vi "Begin.vi"() -> (0 "error out":errorcluster)   [LabVIEW 2013]
doc: "Called before other user functions, this VI is expected to open initial I/O refnums, load in file data, and do all program initialization. Notice that the <B>error out</B> terminal is simply used for data flow. Wiring it to other structures or subVIs ensures that this VI runs first."
uses:
  <vilib>/Rock Robotics/WPI/Joystick/WPI_JoystickDeviceEnum.ctl
  <vilib>/Rock Robotics/SystemInterfaces/Typedef/FPGA_TypedefDigitalModule.ctl
  <vilib>/Rock Robotics/SystemInterfaces/DIO/FPGA_DIOChannel.ctl
  <vilib>/Rock Robotics/SystemInterfaces/DIO/FPGA_DIORelayChannel.ctl
  <vilib>/Rock Robotics/SystemInterfaces/Typedef/FPGA_TypedefSolenoidModule.ctl
  <vilib>/Rock Robotics/WPI/Solenoid/WPI_SolenoidChannel.ctl
  <vilib>/Rock Robotics/SystemInterfaces/DIO/FPGA_DIOPWMChannel.ctl
  <vilib>/Rock Robotics/WPI/Encoder/WPI_EncoderType.ctl
  <vilib>/Rock Robotics/WPI/Solenoid/WPI_SolenoidValue.ctl
  <vilib>/Rock Robotics/WPI/Camera/WPI_CameraImageSize.ctl
  <vilib>/Rock Robotics/WPI/Camera/WPI_CameraWhite Balance Values.ctl
  <vilib>/Rock Robotics/WPI/Camera/WPI_CameraExposure Values.ctl
  <vilib>/Rock Robotics/WPI/Camera/WPI_CameraFrameRate.ctl
  <vilib>/Rock Robotics/WPI/Solenoid/WPI_SolenoidOpenDouble.vi
  <vilib>/Rock Robotics/WPI/Solenoid/WPI_SolenoidSetEnum.vi
  <vilib>/Rock Robotics/WPI/Counter/WPI_CounterDigitalInputToDigitalSource.vi
  <vilib>/Rock Robotics/WPI/RobotDrive/WPI_RobotDriveOpen2MotorWithVictor.vi
  <vilib>/Rock Robotics/WPI/MotorControl/WPI_MotorControlOpen Jaguar.vi
  <vilib>/Rock Robotics/WPI/MotorControl/WPI_MotorControlOpen Victor.vi
  <vilib>/Rock Robotics/WPI/Compressor/WPI_CompressorGetSetRefNum.vi
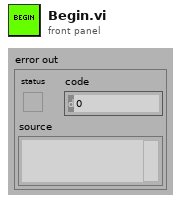
[diagram p1: front panel]
types:
  T1 = typedef "WPI_SolenoidValue.ctl" = enum16{"Off", "On", "Forward", "Reverse"}
  T2 = typedef "FPGA_DIOChannel.ctl" = enum8{"DIO 1", "DIO 2", "DIO 3", "DIO 4", "DIO 5", "DIO 6", "DIO 7", "DIO 8", "DIO 9", "DIO 10", "DIO 11", "DIO 12", "DIO 13", "DIO 14", "Invalid"}
  T3 = typedef "WPI_SolenoidChannel.ctl" = enum8{"Solenoid 1", "Solenoid 2", "Solenoid 3", "Solenoid 4", "Solenoid 5", "Solenoid 6", "Solenoid 7", "Solenoid 8", "Invalid"}
  T4 = typedef "FPGA_DIOPWMChannel.ctl" = enum8{"PWM 1", "PWM 2", "PWM 3", "PWM 4", "PWM 5", "PWM 6", "PWM 7", "PWM 8", "PWM 9", "PWM 10", "Invalid"}
  T5 = typedef "WPI_EncoderType.ctl" = enum16{"1x", "2x", "4x"}
  T6 = typedef "FPGA_TypedefSolenoidModule.ctl" = enum16{"Solenoid Module 1", "Solenoid Module 2"}
  T7 = typedef "FPGA_DIORelayChannel.ctl" = enum8{"Relay 1", "Relay 2", "Relay 3", "Relay 4", "Relay 5", "Relay 6", "Relay 7", "Relay 8", "Invalid"}
  T8 = typedef "WPI_JoystickDeviceEnum.ctl" = enum16{"USB 1", "USB 2", "USB 3", "USB 4", "Kinect 1", "Kinect 2"}
  T9 = typedef "FPGA_TypedefDigitalModule.ctl" = enum16{"Digital Module 1", "Digital Module 2"}
  T10 = typedef "WPI_CameraFrameRate.ctl" = u32
  T11 = typedef "WPI_CameraExposure Values.ctl" = enum16{"Auto", "Flicker-free 50 Hz", "Flicker-free 60 Hz", "Hold current"}
  T12 = typedef "WPI_CameraWhite Balance Values.ctl" = enum16{"Auto", "Fixed indoor", "Fixed outdoor 1", "Fixed outdoor 2", "Fixed fluorescent 1", "Fixed fluorescent 2", "Hold current"}
  T13 = typedef "WPI_CameraImageSize.ctl" = enum16{"640x480", "320x240", "160x120"}
  T14 = typedef "WPI_CameraDevRef.ctl" = cluster{"Camera Address":string, "CameraStatus":errorcluster, "Acquire Image Notifier":refnum<notifier>}
  T15 = typedef "WPI_DigitalInputDevRef.ctl" = cluster{"DevStatus":errorcluster, "DIO Channel":T2, "Digital Module":T9}
  T16 = typedef "WPI_MotorControlDeviceRef.ctl" = cluster{"DeviceStatus":errorcluster, "Type":enum16{"PWM", "CAN"}, "PWM":cluster{"Digital Module":T9, "PWM Channel":T4, "DeadBand":T17}, "CAN":cluster{"Device Number":u8, "Control Mode":T18, "Semaphore":T19, "Max Vout":dbl}, "Invert":bool, "TransformRef":T20, "InvTransformRef":T20}
  T17 = typedef "WPI_PWMDeadband.ctl" = cluster{"Name":string, "maxPositivePwm":i32, "minPositivePwm":i32, "centerPwm":i32, "maxNegativePwm":i32, "minNegativePwm":i32, "angularRange":u16}
  T18 = typedef "WPI_CANJaguar_ControlMode.ctl" = enum8{"Percent VBus", "Current", "Speed", "Position", "Voltage"}
  T19 = typedef "Semaphore RefNum" = refnum<k1>
  T20 = typedef "WPI_PWMTransform_ConPane.ctl" = refnum<vi>
  T21 = typedef "WPI_SolenoidDevRef.ctl" = cluster{"DevStatus":errorcluster, "Solenoid Module":T6, "Forward Solenoid Channel":T3, "Reverse Solenoid Channel":T3}
  T22 = typedef "FPGA_CounterEncoderSourceConvertionLVSourceType.ctl" = cluster{"DevStatus":errorcluster, "AnalogTriggerMode?":bool, "DigitalMode":cluster{"Digital Module":T9, "DIO Channel":T23}, "AnalogTriggerMode":cluster{"AnalogTriggerIndex":T24, "OutputType":T25}}
  T23 = typedef "FPGA_DIODigitalSourceChannel.ctl" = enum8{"DIO 1", "DIO 2", "DIO 3", "DIO 4", "DIO 5", "DIO 6", "DIO 7", "DIO 8", "DIO 9", "DIO 10", "DIO 11", "DIO 12", "DIO 13", "DIO 14", "Disabled"}
  T24 = typedef "FPGA_AnalogTriggerIndex.ctl" = enum8{"Trig 0", "Trig 1", "Trig 2", "Trig 3", "Trig 4", "Trig 5", "Trig 6", "Trig 7", "Invalid"}
  T25 = typedef "FPGA_AnalogTriggerOutType.ctl" = enum16{"InWindow", "TriggerState", "Rising", "Falling"}
  T26 = typedef "WPI_CompressorDevRef.ctl" = cluster{"DevStatus":errorcluster, "DigitalInputDevRef":T15, "RelayDevRef":T27}
  T27 = typedef "WPI_RelayDevRef.ctl" = cluster{"DevStatus":errorcluster, "Relay Channel":T7, "Digital Module":T9, "Relay Direction":T28}
  T28 = typedef "WPI_RelayDirection.ctl" = enum16{"Both directions", "Forward only", "Reverse only"}
  T29 = typedef "WPI_RobotDriveDevRef.ctl" = cluster{"DevStatus":errorcluster, "Motors[]":T16[], "Square Inputs":bool, "Max Output":dbl, "Isochronous":bool}
  T30 = typedef "WPI_EncoderDevRef.ctl" = cluster{"DevStatus":errorcluster, "EncoderIndex":T31, "CounterIndex":T32, "DistancePerCount":dbl, "Decoding Type":T5}
  T31 = typedef "FPGA_EncoderIdx.ctl" = enum8{"Enc 0", "Enc 1", "Enc 2", "Enc 3", "Invalid"}
  T32 = typedef "FPGA_CounterCtrSystemIndex.ctl" = enum8{"Ctr 0", "Ctr 1", "Ctr 2", "Ctr 3", "Ctr 4", "Ctr 5", "Ctr 6", "Ctr 7", "Invalid"}
  T33 = typedef "WPI_JoystickDevRef.ctl" = cluster{"Device":T8}
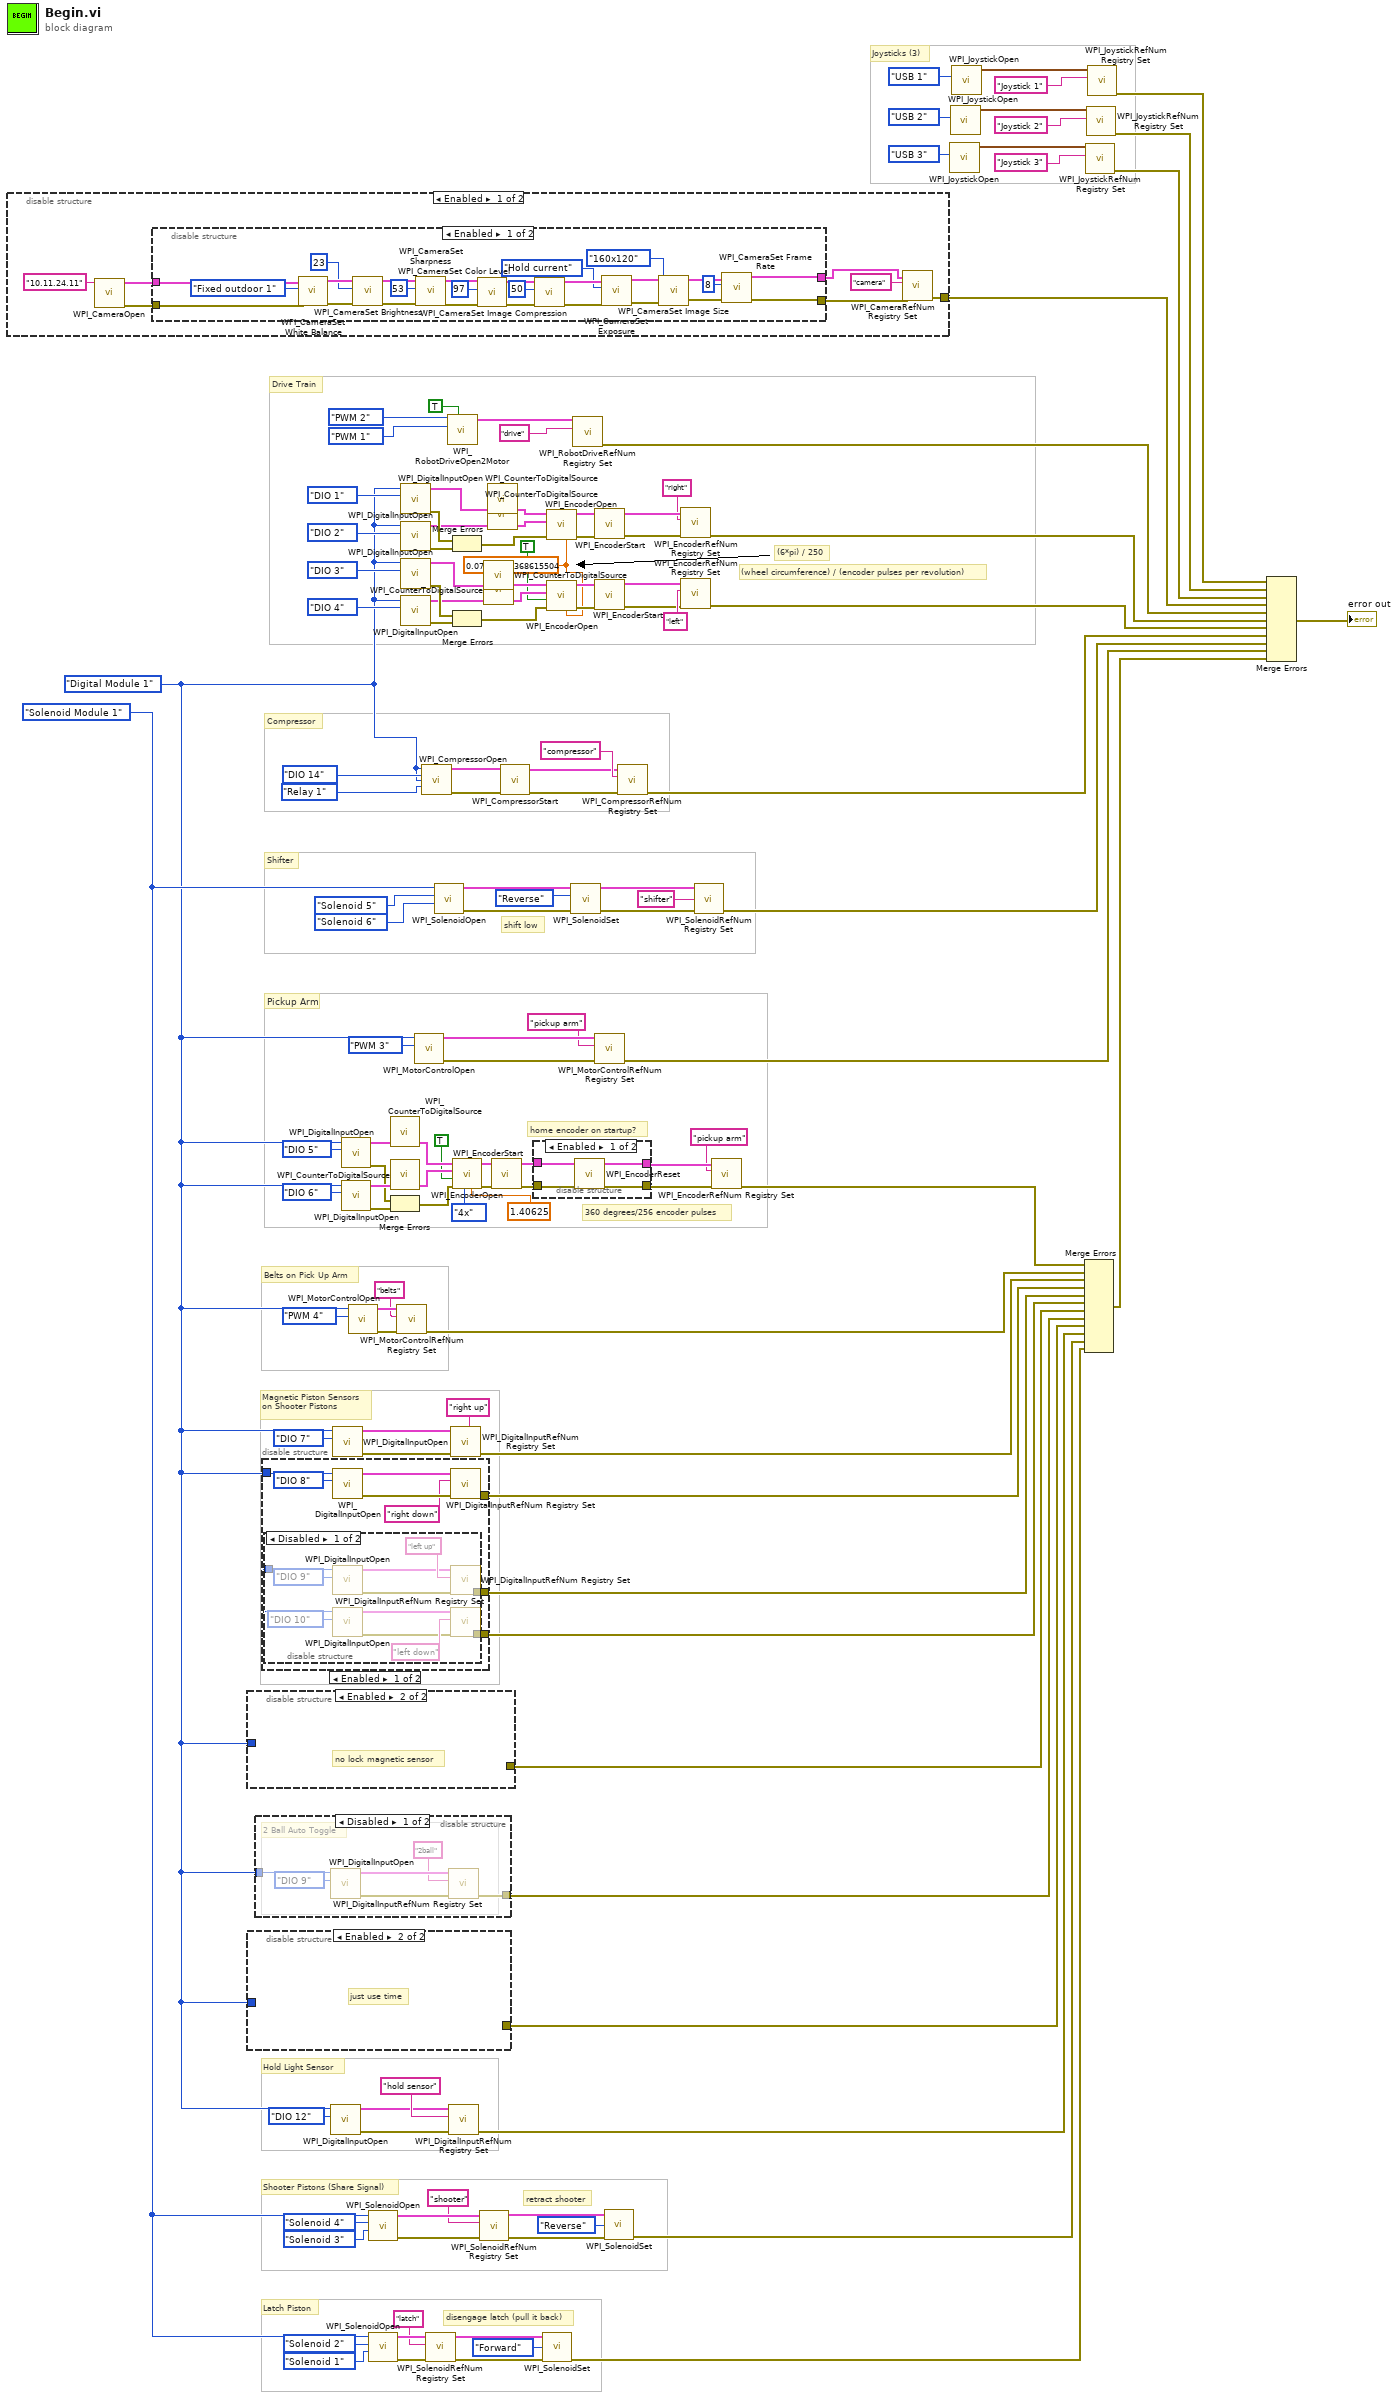
[diagram p0: block diagram]
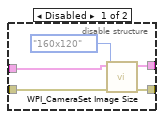
[diagram p4: hidden frame]
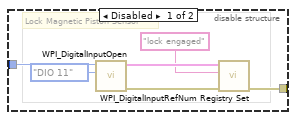
[diagram p6: hidden frame]
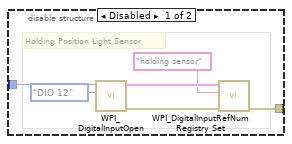
[diagram p9: hidden frame]
diagram:
  w80 = 0.07539822368615504 ("DistancePerCount")
  w23 = FPGA_TypedefSolenoidModule."Solenoid Module 1" ("Solenoid Module (Module 1)")
  w12 = FPGA_TypedefDigitalModule."Digital Module 1" ("Digital Module (Module 1)")
  # "retract shooter"
  # "disengage latch (pull it back)"
  # "360 degrees/256 encoder pulses"
  # "Hold Light Sensor"
  # "Joysticks (3)"
  # "Latch Piston"
  # "Shooter Pistons (Share Signal)"
  # "Magnetic Piston Sensors\non Shooter Pistons"
  # "Belts on Pick Up Arm"
  # "Pickup Arm"
  # "home encoder on startup?"
  # "Shifter"
  # "Compressor"
  # "Drive Train"
  # "shift low"
  # "(wheel circumference) / (encoder pulses per revolution)"
  # "(6*pi) / 250"
  n1 = disable-structure shown="Enabled" {
    disable-tunnel: [w143 _] -> w124
    frame Enabled {
      n2 = call <vilib>:"WPI_CameraOpen.vi"("Camera Address"="10.11.24.11") -> ("error out"=w138:errorcluster, "CameraDevRef"=w140:T14)  [unwired: 9 in]
      n3 = disable-structure shown="Enabled" {
        disable-tunnel: w140 -> [w167 w173]
        disable-tunnel: [w145 w172] -> w139
        disable-tunnel: w138 -> [w154 w171]
        disable-tunnel: [w144 w170] -> w137
        frame Enabled {
          n4 = call <vilib>:"WPI_CameraSet White Balance.vi"("error in (no error)"=w154, "White Balance"=WPI_CameraWhite_Balance_Values."Fixed outdoor 1", "CameraDevRef"=w167) -> ("error out"=w155:errorcluster, "CameraDevRef Out"=w166:T14)  [unwired: 7 in]
          n5 = call <vilib>:"WPI_CameraSet Brightness.vi"("error in (no error)"=w155, "Brightness"=23, "CameraDevRef"=w166) -> ("error out"=w156:errorcluster, "CameraDevRef Out"=w165:T14)  [unwired: 7 in]
          n6 = call <vilib>:"WPI_CameraSet Sharpness.vi"("error in (no error)"=w156, "Sharpness"=53, "CameraDevRef"=w165) -> ("error out"=w157:errorcluster, "CameraDevRef Out"=w164:T14)  [unwired: 7 in]
          n7 = call <vilib>:"WPI_CameraSet Color Level.vi"("error in (no error)"=w157, "Color Level"=97, "CameraDevRef"=w164) -> ("error out"=w158:errorcluster, "CameraDevRef Out"=w163:T14)  [unwired: 7 in]
          n8 = call <vilib>:"WPI_CameraSet Image Compression.vi"("error in (no error)"=w158, "Compression"=50, "CameraDevRef"=w163) -> ("error out"=w169:errorcluster, "CameraDevRef Out"=w168:T14)  [unwired: 7 in]
          n9 = call <vilib>:"WPI_CameraSet Exposure.vi"("error in (no error)"=w169, "Exposure"=WPI_CameraExposure_Values."Hold current", "CameraDevRef"=w168) -> ("error out"=w159:errorcluster, "CameraDevRef Out"=w162:T14)  [unwired: 7 in]
          n10 = call <vilib>:"WPI_CameraSet Image Size.vi"("error in (no error)"=w159, "Image Size"=WPI_CameraImageSize."160x120", "CameraDevRef"=w162) -> ("error out"=w160:errorcluster, "CameraDevRef Out"=w161:T14)  [unwired: 7 in]
          n11 = call <vilib>:"WPI_CameraSet Frame Rate.vi"("error in (no error)"=w160, "Frame Rate (fps)"=T10 8, "CameraDevRef"=w161) -> ("error out"=w144:errorcluster, "CameraDevRef Out"=w145:T14)  [unwired: 7 in]
        }
        frame Disabled {
          n12 = disable-structure shown="Enabled" {
            disable-tunnel: w171 -> [w177 w179]
            disable-tunnel: [w176 w179] -> w170
            disable-tunnel: w173 -> [w175 w180]
            disable-tunnel: [w174 w180] -> w172
            frame Disabled {
              n13 = call <vilib>:"WPI_CameraSet Image Size.vi"("error in (no error)"=w177, "Image Size"=WPI_CameraImageSize."160x120", "CameraDevRef"=w175) -> ("error out"=w176:errorcluster, "CameraDevRef Out"=w174:T14)  [unwired: 7 in]
            }
            frame Enabled {
            }
          }
        }
      }
      n14 = call <vilib>:"WPI_CameraRefNum Registry Set.vi"("error in (no error)"=w137, "refnum name"="camera", "CameraDevRef"=w139) -> ("error out"=w143:errorcluster)  [unwired: 7 in, 1 out]
    }
    frame Disabled {
    }
  }
  n15 = disable-structure shown="Enabled" {
    disable-tunnel: w12 -> [w182 _]
    disable-tunnel: [w181 _] -> w16
    frame Disabled {
      # "Lock Magnetic Piston Sensor"
      n16 = call <vilib>:"WPI_DigitalInputOpen.vi"("DIO Channel"=FPGA_DIOChannel."DIO 11", "Digital Module (Module 1)"=w182) -> ("error out"=w185:errorcluster, "DigitalInputDevRef"=w184:T15)  [unwired: 8 in]
      n17 = call <vilib>:"WPI_DigitalInputRefNum Registry Set.vi"("error in (no error)"=w185, "refnum name"="lock engaged", "DigitalInputDevRef"=w184) -> ("error out"=w181:errorcluster)  [unwired: 7 in, 1 out]
    }
    frame Enabled {
      # "no lock magnetic sensor"
    }
  }
  n18 = disable-structure shown="Enabled" {
    disable-tunnel: w12 -> [w188 _]
    disable-tunnel: [w187 _] -> w9
    frame Disabled {
      # "Holding Position Light Sensor"
      n19 = call <vilib>:"WPI_DigitalInputOpen.vi"("DIO Channel"=FPGA_DIOChannel."DIO 12", "Digital Module (Module 1)"=w188) -> ("error out"=w191:errorcluster, "DigitalInputDevRef"=w190:T15)  [unwired: 8 in]
      n20 = call <vilib>:"WPI_DigitalInputRefNum Registry Set.vi"("error in (no error)"=w191, "refnum name"="holding sensor", "DigitalInputDevRef"=w190) -> ("error out"=w187:errorcluster)  [unwired: 7 in, 1 out]
    }
    frame Enabled {
      # "just use time"
    }
  }
  n21 = disable-structure shown="Disabled" {
    disable-tunnel: w12 -> [w198 _]
    disable-tunnel: [w193 _] -> w8
    frame Disabled {
      # "2 Ball Auto Toggle"
      n22 = call <vilib>:"WPI_DigitalInputOpen.vi"("DIO Channel"=FPGA_DIOChannel."DIO 9", "Digital Module (Module 1)"=w198) -> ("error out"=w196:errorcluster, "DigitalInputDevRef"=w195:T15)  [unwired: 8 in]
      n23 = call <vilib>:"WPI_DigitalInputRefNum Registry Set.vi"("error in (no error)"=w196, "refnum name"="2ball", "DigitalInputDevRef"=w195) -> ("error out"=w193:errorcluster)  [unwired: 7 in, 1 out]
    }
    frame Enabled {
    }
  }
  n24 = disable-structure shown="Enabled" {
    disable-tunnel: [w203 _] -> w34
    disable-tunnel: w12 -> [w201 _]
    disable-tunnel: [w200 _] -> w18
    disable-tunnel: [w199 _] -> w17
    frame Enabled {
      n25 = disable-structure shown="Disabled" {
        disable-tunnel: w201 -> [w209 _]
        disable-tunnel: [w208 _] -> w200
        disable-tunnel: [w207 _] -> w199
        frame Disabled {
          n26 = call <vilib>:"WPI_DigitalInputOpen.vi"("DIO Channel"=FPGA_DIOChannel."DIO 9", "Digital Module (Module 1)"=w209) -> ("error out"=w210:errorcluster, "DigitalInputDevRef"=w211:T15)  [unwired: 8 in]
          n27 = call <vilib>:"WPI_DigitalInputOpen.vi"("DIO Channel"=FPGA_DIOChannel."DIO 10", "Digital Module (Module 1)"=w209) -> ("error out"=w212:errorcluster, "DigitalInputDevRef"=w213:T15)  [unwired: 8 in]
          n28 = call <vilib>:"WPI_DigitalInputRefNum Registry Set.vi"("error in (no error)"=w210, "refnum name"="left up", "DigitalInputDevRef"=w211) -> ("error out"=w208:errorcluster)  [unwired: 7 in, 1 out]
          n29 = call <vilib>:"WPI_DigitalInputRefNum Registry Set.vi"("error in (no error)"=w212, "refnum name"="left down", "DigitalInputDevRef"=w213) -> ("error out"=w207:errorcluster)  [unwired: 7 in, 1 out]
        }
        frame Enabled {
        }
      }
      n30 = call <vilib>:"WPI_DigitalInputOpen.vi"("DIO Channel"=FPGA_DIOChannel."DIO 8", "Digital Module (Module 1)"=w201) -> ("error out"=w206:errorcluster, "DigitalInputDevRef"=w205:T15)  [unwired: 8 in]
      n31 = call <vilib>:"WPI_DigitalInputRefNum Registry Set.vi"("error in (no error)"=w206, "refnum name"="right down", "DigitalInputDevRef"=w205) -> ("error out"=w203:errorcluster)  [unwired: 7 in, 1 out]
    }
    frame Disabled {
      # "dang, only one sensor\non the pistons..."
    }
  }
  n32 = call <vilib>:"WPI_DigitalInputOpen.vi"("DIO Channel"=FPGA_DIOChannel."DIO 12", "Digital Module (Module 1)"=w12) -> ("error out"=w20:errorcluster, "DigitalInputDevRef"=w21:T15)  [unwired: 8 in]
  n33 = call <vilib>:"WPI_DigitalInputOpen.vi"("DIO Channel"=FPGA_DIOChannel."DIO 7", "Digital Module (Module 1)"=w12) -> ("error out"=w39:errorcluster, "DigitalInputDevRef"=w38:T15)  [unwired: 8 in]
  n34 = call <vilib>:"WPI_DigitalInputOpen.vi"("DIO Channel"=FPGA_DIOChannel."DIO 5", "Digital Module (Module 1)"=w12) -> ("error out"=w56:errorcluster, "DigitalInputDevRef"=w61:T15)  [unwired: 8 in]
  n35 = call <vilib>:"WPI_DigitalInputOpen.vi"("DIO Channel"=FPGA_DIOChannel."DIO 6", "Digital Module (Module 1)"=w12) -> ("error out"=w57:errorcluster, "DigitalInputDevRef"=w60:T15)  [unwired: 8 in]
  n36 = call-poly <vilib>:"WPI_MotorControlOpen.vi"("PWM Channel"=FPGA_DIOPWMChannel."PWM 4", "Digital Module (Module 1)"=w12) -> ("error out"=w45:errorcluster, "MotorControlDeviceRef"=w44:T16)  [unwired: 8 in]
  n37 = call-poly <vilib>:"WPI_SolenoidOpen.vi"("Reverse Solenoid Channel"=WPI_SolenoidChannel."Solenoid 3", "Forward Solenoid Channel"=WPI_SolenoidChannel."Solenoid 4", "Solenoid Module (Module 1)"=w23) -> ("error out"=w29:errorcluster, "SolenoidDevRef"=w28:T21)  [unwired: 7 in]
  n38 = call-poly <vilib>:"WPI_SolenoidOpen.vi"("Reverse Solenoid Channel"=WPI_SolenoidChannel."Solenoid 1", "Forward Solenoid Channel"=WPI_SolenoidChannel."Solenoid 2", "Solenoid Module (Module 1)"=w23) -> ("error out"=w27:errorcluster, "SolenoidDevRef"=w26:T21)  [unwired: 7 in]
  n39 = call-poly <vilib>:"WPI_CounterToDigitalSource.vi"("DigitalInputDevRef"=w61) -> ("Digital Source"=w59:T22)  [unwired: 6 in]
  n40 = call-poly <vilib>:"WPI_CounterToDigitalSource.vi"("DigitalInputDevRef"=w60) -> ("Digital Source"=w58:T22)  [unwired: 6 in]
  n41 = Merge Errors(w56, w57) -> (w55:errorcluster)
  n42 = call <vilib>:"WPI_MotorControlRefNum Registry Set.vi"("error in (no error)"=w45, "refnum name"="belts", "MotorControlDevRef"=w44) -> ("error out"=w42:errorcluster)  [unwired: 7 in, 1 out]
  n43 = call <vilib>:"WPI_DigitalInputOpen.vi"("DIO Channel"=FPGA_DIOChannel."DIO 1", "Digital Module (Module 1)"=w12) -> ("error out"=w74:errorcluster, "DigitalInputDevRef"=w88:T15)  [unwired: 8 in]
  n44 = call <vilib>:"WPI_DigitalInputOpen.vi"("DIO Channel"=FPGA_DIOChannel."DIO 2", "Digital Module (Module 1)"=w12) -> ("error out"=w76:errorcluster, "DigitalInputDevRef"=w73:T15)  [unwired: 8 in]
  n45 = call <vilib>:"WPI_DigitalInputOpen.vi"("DIO Channel"=FPGA_DIOChannel."DIO 3", "Digital Module (Module 1)"=w12) -> ("error out"=w77:errorcluster, "DigitalInputDevRef"=w102:T15)  [unwired: 8 in]
  n46 = call <vilib>:"WPI_DigitalInputOpen.vi"("DIO Channel"=FPGA_DIOChannel."DIO 4", "Digital Module (Module 1)"=w12) -> ("error out"=w79:errorcluster, "DigitalInputDevRef"=w72:T15)  [unwired: 8 in]
  n47 = call-poly <vilib>:"WPI_MotorControlOpen.vi"("PWM Channel"=FPGA_DIOPWMChannel."PWM 3", "Digital Module (Module 1)"=w12) -> ("error out"=w68:errorcluster, "MotorControlDeviceRef"=w67:T16)  [unwired: 8 in]
  n48 = call <vilib>:"WPI_CompressorOpen.vi"("Pressure Switch Digital Module (Module 1)"=w12, "Pressure Switch DIO Channel"=FPGA_DIOChannel."DIO 14", "Relay Digital Module (Module 1)"=w12, "Relay Channel"=FPGA_DIORelayChannel."Relay 1") -> ("CompressorDevRef"=w116:T26, "error out"=w115:errorcluster)  [unwired: 10 in]
  n49 = call <vilib>:"WPI_SolenoidRefNum Registry Set.vi"("error in (no error)"=w27, "refnum name"="latch", "SolenoidDevRef"=w26) -> ("error out"=w14:errorcluster, "SolenoidDevRef"=w13:T21)  [unwired: 7 in]
  n50 = call-poly <vilib>:"WPI_SolenoidOpen.vi"("Reverse Solenoid Channel"=WPI_SolenoidChannel."Solenoid 6", "Forward Solenoid Channel"=WPI_SolenoidChannel."Solenoid 5", "Solenoid Module (Module 1)"=w23) -> ("error out"=w107:errorcluster, "SolenoidDevRef"=w108:T21)  [unwired: 7 in]
  n51 = call-poly <vilib>:"WPI_RobotDriveOpen2Motor.vi"("Left Motor Inverted"=TRUE, "Right Motor"=FPGA_DIOPWMChannel."PWM 1", "Left Motor"=FPGA_DIOPWMChannel."PWM 2") -> ("RobotDriveDevRef"=w104:T29)  [unwired: 7 in, 1 out]
  n52 = call <vilib>:"WPI_DigitalInputRefNum Registry Set.vi"("error in (no error)"=w20, "refnum name"="hold sensor", "DigitalInputDevRef"=w21) -> ("error out"=w10:errorcluster)  [unwired: 7 in, 1 out]
  n53 = call <vilib>:"WPI_DigitalInputRefNum Registry Set.vi"("error in (no error)"=w39, "refnum name"="right up", "DigitalInputDevRef"=w38) -> ("error out"=w35:errorcluster)  [unwired: 7 in, 1 out]
  n54 = Merge Errors(w74, w76) -> (w75:errorcluster)
  n55 = Merge Errors(w77, w79) -> (w78:errorcluster)
  n56 = call <vilib>:"WPI_EncoderOpen.vi"("DistancePerCount"=1.40625, "Decoding Type"=WPI_EncoderType."4x", "error in (no error)"=w55, "Invert Direction (False)"=TRUE, "BSource"=w58, "ASource"=w59) -> ("error out"=w54:errorcluster, "EncoderDevRef"=w53:T30)  [unwired: 4 in]
  n57 = call <vilib>:"WPI_SolenoidRefNum Registry Set.vi"("error in (no error)"=w29, "refnum name"="shooter", "SolenoidDevRef"=w28) -> ("error out"=w4:errorcluster, "SolenoidDevRef"=w5:T21)  [unwired: 7 in]
  n58 = call-poly <vilib>:"WPI_CounterToDigitalSource.vi"("DigitalInputDevRef"=w102) -> ("Digital Source"=w95:T22)  [unwired: 6 in]
  n59 = call-poly <vilib>:"WPI_CounterToDigitalSource.vi"("DigitalInputDevRef"=w72) -> ("Digital Source"=w96:T22)  [unwired: 6 in]
  n60 = call-poly <vilib>:"WPI_CounterToDigitalSource.vi"("DigitalInputDevRef"=w88) -> ("Digital Source"=w94:T22)  [unwired: 6 in]
  n61 = call-poly <vilib>:"WPI_CounterToDigitalSource.vi"("DigitalInputDevRef"=w73) -> ("Digital Source"=w93:T22)  [unwired: 6 in]
  n62 = call <vilib>:"WPI_EncoderStart.vi"("error in (no error)"=w54, "EncoderDevRef"=w53) -> ("error out"=w52:errorcluster, "EncoderDevRef"=w51:T30)  [unwired: 8 in]
  n63 = call <vilib>:"WPI_CompressorStart.vi"("error in (no error)"=w115, "CompressorDevRef"=w116) -> ("error out"=w114:errorcluster, "CompressorDevRef"=w113:T26)  [unwired: 8 in]
  n64 = disable-structure shown="Enabled" {
    disable-tunnel: w52 -> [w221 w222]
    disable-tunnel: w51 -> [w220 w223]
    disable-tunnel: [w219 w223] -> w49
    disable-tunnel: [w218 w222] -> w50
    frame Enabled {
      n65 = call <vilib>:"WPI_EncoderReset.vi"("error in (no error)"=w221, "EncoderDevRef"=w220) -> ("error out"=w218:errorcluster, "EncoderDevRef"=w219:T30)  [unwired: 8 in]
    }
    frame Disabled {
    }
  }
  n66 = call-poly <vilib>:"WPI_SolenoidSet.vi"("error in (no error)"=w14, "Value"=WPI_SolenoidValue."Forward", "SolenoidDevRef"=w13) -> ("error out"=w11:errorcluster)  [unwired: 7 in, 1 out]
  n67 = call <vilib>:"WPI_EncoderOpen.vi"("DistancePerCount"=w80, "error in (no error)"=w75, "BSource"=w93, "ASource"=w94) -> ("error out"=w92:errorcluster, "EncoderDevRef"=w91:T30)  [unwired: 6 in]
  n68 = call <vilib>:"WPI_EncoderOpen.vi"("DistancePerCount"=w80, "error in (no error)"=w78, "Invert Direction (False)"=TRUE, "BSource"=w96, "ASource"=w95) -> ("error out"=w97:errorcluster, "EncoderDevRef"=w98:T30)  [unwired: 5 in]
  n69 = call-poly <vilib>:"WPI_SolenoidSet.vi"("error in (no error)"=w107, "Value"=WPI_SolenoidValue."Reverse", "SolenoidDevRef"=w108) -> ("error out"=w106:errorcluster, "SolenoidDevRef"=w105:T21)  [unwired: 7 in]
  n70 = call <vilib>:"WPI_RobotDriveRefNum Registry Set.vi"("refnum name"="drive", "RobotDriveDevRef"=w104) -> ("error out"=w123:errorcluster)  [unwired: 8 in, 1 out]
  n71 = call <vilib>:"WPI_EncoderStart.vi"("error in (no error)"=w92, "EncoderDevRef"=w91) -> ("error out"=w90:errorcluster, "EncoderDevRef"=w89:T30)  [unwired: 8 in]
  n72 = call <vilib>:"WPI_EncoderStart.vi"("error in (no error)"=w97, "EncoderDevRef"=w98) -> ("error out"=w99:errorcluster, "EncoderDevRef"=w100:T30)  [unwired: 8 in]
  n73 = call <vilib>:"WPI_MotorControlRefNum Registry Set.vi"("error in (no error)"=w68, "refnum name"="pickup arm", "MotorControlDevRef"=w67) -> ("error out"=w64:errorcluster)  [unwired: 7 in, 1 out]
  n74 = call-poly <vilib>:"WPI_SolenoidSet.vi"("error in (no error)"=w4, "Value"=WPI_SolenoidValue."Reverse", "SolenoidDevRef"=w5) -> ("error out"=w3:errorcluster)  [unwired: 7 in, 1 out]
  n75 = call <vilib>:"WPI_CompressorRefNum Registry Set.vi"("error in (no error)"=w114, "refnum name"="compressor", "CompressorDevRef"=w113) -> ("error out"=w69:errorcluster)  [unwired: 7 in, 1 out]
  n76 = call <vilib>:"WPI_EncoderRefNum Registry Set.vi"("error in (no error)"=w90, "refnum name"="right", "EncoderDevRef"=w89) -> ("error out"=w122:errorcluster)  [unwired: 7 in, 1 out]
  n77 = call <vilib>:"WPI_EncoderRefNum Registry Set.vi"("error in (no error)"=w99, "refnum name"="left", "EncoderDevRef"=w100) -> ("error out"=w121:errorcluster)  [unwired: 7 in, 1 out]
  n78 = call <vilib>:"WPI_SolenoidRefNum Registry Set.vi"("error in (no error)"=w106, "refnum name"="shifter", "SolenoidDevRef"=w105) -> ("error out"=w70:errorcluster)  [unwired: 7 in, 1 out]
  n79 = call <vilib>:"WPI_EncoderRefNum Registry Set.vi"("error in (no error)"=w50, "refnum name"="pickup arm", "EncoderDevRef"=w49) -> ("error out"=w41:errorcluster)  [unwired: 7 in, 1 out]
  n80 = call <vilib>:"WPI_JoystickOpen.vi"("JoystickDevice"=WPI_JoystickDeviceEnum."USB 3") -> ("JoystickDevRef"=w135:T33)  [unwired: 10 in]
  n81 = call <vilib>:"WPI_JoystickOpen.vi"("JoystickDevice"=WPI_JoystickDeviceEnum."USB 2") -> ("JoystickDevRef"=w132:T33)  [unwired: 10 in]
  n82 = call <vilib>:"WPI_JoystickOpen.vi"("JoystickDevice"=WPI_JoystickDeviceEnum."USB 1") -> ("JoystickDevRef"=w129:T33)  [unwired: 10 in]
  n83 = Merge Errors(w41, w42, w35, w34, w18, w17, w16, w8, w9, w10, w3, w11) -> (w40:errorcluster)
  n84 = call <vilib>:"WPI_JoystickRefNum Registry Set.vi"("refnum name"="Joystick 3", "JoystickDevRef"=w135) -> ("error out"=w125:errorcluster)  [unwired: 8 in, 1 out]
  n85 = call <vilib>:"WPI_JoystickRefNum Registry Set.vi"("refnum name"="Joystick 2", "JoystickDevRef"=w132) -> ("error out"=w126:errorcluster)  [unwired: 8 in, 1 out]
  n86 = call <vilib>:"WPI_JoystickRefNum Registry Set.vi"("refnum name"="Joystick 1", "JoystickDevRef"=w129) -> ("error out"=w127:errorcluster)  [unwired: 8 in, 1 out]
  n87 = Merge Errors(w127, w126, w125, w124, w123, w122, w121, w69, w70, w64, w40) -> (→"error out":errorcluster)
